vi "test_read_AB2504.vi"() -> ()   [LabVIEW 2015, in "Tausand AB1000.lvlib"]
uses:
  <instrlib>/Tausand AB1000/Tausand AB1000.lvlib
  <instrlib>/Tausand AB1000/Public/Controls/settings4ch.ctl
  <instrlib>/Tausand AB1000/Public/Controls/configMultipleCoincRing.ctl
  <instrlib>/Tausand AB1000/Public/Controls/counters4ch.ctl
  <instrlib>/Tausand AB1000/Public/Controls/deviceTypeRing.ctl
  <instrlib>/Tausand AB1000/Public/Controls/serialCommand.ctl
  <vilib>/Instr/_visa.llb/VISA Configure Serial Port (Instr).vi
panel:
  out "mode 3 timer":dbl format="%.1p"
  out "AB settg read timer":dbl format="%.1p"
  out "AB data read timer":dbl format="%.1p"
  out "porcentaje mal":dbl(slide) scale=0.0..100.0
  in  "ABlib on?":bool
  out "mode 2 timer":dbl format="%.1p"
  in  "mode3 on?":bool
  in  "mode2 on?":bool
  out "mode3 addr":u8[](array[numeric]) format="%.0x"
  out "mode3 data":u32[](array[numeric]) format="%.0x"
  in  "VISA resource name":refnum<visa-resource-name>
  in  "baud rate (115200)":u32=115200
  out "error out":errorcluster
  in  "device type":T1=1504 items=["any"=0, "AB1002"=1002, "AB1004"=1004, "AB1502"=1502, "AB1504"=1504, "AB1902"=1902, "AB1904"=1904]
  out "ID out":u32
  out "checksum ok?":bool
  in  "stop":bool
  out "porcentaje ok":dbl(slide) scale=0.0..100.0
  out "time left ms out":u32
  out "total ok":i32
  out "total try":i32
  out "output cluster 4ch":T2
  out "output cluster settings 4ch":T3 {"config_multiple_1" items=["ABC"=224, "ABD"=208, "ACD"=176, "BCD"=112, "ABCD"=240]; "sleep_D" max=100 step=5; "sleep_C" max=100 step=5; "sleep_B" max=100 step=5; "sleep_A" max=100 step=5; "delay_D" max=100 step=5; "delay_C" max=100 step=5; "delay_B" max=100 step=5; "delay_A" max=100 step=5; "coincidence_window" min=5 max=10000 step=5; "sampling" items=["1ms"=1, "2ms"=2, "3ms"=3, "4ms"=4, "5ms"=5, "6ms"=6, "7ms"=7, "8ms"=8, "9ms"=9, "10ms"=10, "11ms"=11, "12ms"=12, "13ms"=13, "14ms"=14, "15ms"=15, "16ms"=16, "17ms"=17, "18ms"=18, "19ms"=19, "20ms"=20, "21ms"=21, "22ms"=22, "23ms"=23, "24ms"=24, "25ms"=25, "26ms"=26, "27ms"=27, "28ms"=28, "29ms"=29, "30ms"=30, "31ms"=31, "32ms"=32, "33ms"=33, "34ms"=34, "35ms"=35, "36ms"=36, "37ms"=37, "38ms"=38, "39ms"=39, "40ms"=40, "41ms"=41, "42ms"=42, "43ms"=43, "44ms"=44, "45ms"=45, "46ms"=46, "47ms"=47, "48ms"=48, "49ms"=49, "50ms"=50, "51ms"=51, "52ms"=52, "53ms"=53, "54ms"=54, "55ms"=55, "56ms"=56, "57ms"=57, "58ms"=58, "59ms"=59, "60ms"=60, "61ms"=61, "62ms"=62, "63ms"=63, "64ms"=64, "65ms"=65, "66ms"=66, "67ms"=67, "68ms"=68, "69ms"=69, "70ms"=70, "71ms"=71, "72ms"=72, "73ms"=73, "74ms"=74, "75ms"=75, "76ms"=76, "77ms"=77, "78ms"=78, "79ms"=79, "80ms"=80, "81ms"=81, "82ms"=82, "83ms"=83, "84ms"=84, "85ms"=85, "86ms"=86, "87ms"=87, "88ms"=88, "89ms"=89, "90ms"=90, "91ms"=91, "92ms"=92, "93ms"=93, "94ms"=94, "95ms"=95, "96ms"=96, "97ms"=97, "98ms"=98, "99ms"=99, "100ms"=100, "110ms"=110, "120ms"=120, "130ms"=130, "140ms"=140, "150ms"=150, "160ms"=160, "170ms"=170, "180ms"=180, "190ms"=190, "200ms"=200, "210ms"=210, "220ms"=220, "230ms"=230, "240ms"=240, "250ms"=250, "260ms"=260, "270ms"=270, "280ms"=280, "290ms"=290, "300ms"=300, "310ms"=310, "320ms"=320, "330ms"=330, "340ms"=340, "350ms"=350, "360ms"=360, "370ms"=370, "380ms"=380, "390ms"=390, "400ms"=400, "410ms"=410, "420ms"=420, "430ms"=430, "440ms"=440, "450ms"=450, "460ms"=460, "470ms"=470, "480ms"=480, "490ms"=490, "500ms"=500, "510ms"=510, "520ms"=520, "530ms"=530, "540ms"=540, "550ms"=550, "560ms"=560, "570ms"=570, "580ms"=580, "590ms"=590, "600ms"=600, "610ms"=610, "620ms"=620, "630ms"=630, "640ms"=640, "650ms"=650, "660ms"=660, "670ms"=670, "680ms"=680, "690ms"=690, "700ms"=700, "710ms"=710, "720ms"=720, "730ms"=730, "740ms"=740, "750ms"=750, "760ms"=760, "770ms"=770, "780ms"=780, "790ms"=790, "800ms"=800, "810ms"=810, "820ms"=820, "830ms"=830, "840ms"=840, "850ms"=850, "860ms"=860, "870ms"=870, "880ms"=880, "890ms"=890, "900ms"=900, "910ms"=910, "920ms"=920, "930ms"=930, "940ms"=940, "950ms"=950, "960ms"=960, "970ms"=970, "980ms"=980, "990ms"=990, "1,0s"=1000, "1,1s"=1100, "1,2s"=1200, "1,3s"=1300, "1,4s"=1400, "1,5s"=1500, "1,6s"=1600, "1,7s"=1700, "1,8s"=1800, "1,9s"=1900, "2,0s"=2000, "2,1s"=2100, "2,2s"=2200, "2,3s"=2300, "2,4s"=2400, "2,5s"=2500, "2,6s"=2600, "2,7s"=2700, "2,8s"=2800, "2,9s"=2900, "3,0s"=3000, "3,1s"=3100, "3,2s"=3200, "3,3s"=3300, "3,4s"=3400, "3,5s"=3500, "3,6s"=3600, "3,7s"=3700, "3,8s"=3800, "3,9s"=3900, "4,0s"=4000, "4,1s"=4100, "4,2s"=4200, "4,3s"=4300, "4,4s"=4400, "4,5s"=4500, "4,6s"=4600, "4,7s"=4700, "4,8s"=4800, "4,9s"=4900, "5,0s"=5000, "5,1s"=5100, "5,2s"=5200, "5,3s"=5300, "5,4s"=5400, "5,5s"=5500, "5,6s"=5600, "5,7s"=5700, "5,8s"=5800, "5,9s"=5900, "6,0s"=6000, "6,1s"=6100, "6,2s"=6200, "6,3s"=6300, "6,4s"=6400, "6,5s"=6500, "6,6s"=6600, "6,7s"=6700, "6,8s"=6800, "6,9s"=6900, "7,0s"=7000, "7,1s"=7100, "7,2s"=7200, "7,3s"=7300, "7,4s"=7400, "7,5s"=7500, "7,6s"=7600, "7,7s"=7700, "7,8s"=7800, "7,9s"=7900, "8,0s"=8000, "8,1s"=8100, "8,2s"=8200, "8,3s"=8300, "8,4s"=8400, "8,5s"=8500, "8,6s"=8600, "8,7s"=8700, "8,8s"=8800, "8,9s"=8900, "9,0s"=9000, "9,1s"=9100, "9,2s"=9200, "9,3s"=9300, "9,4s"=9400, "9,5s"=9500, "9,6s"=9600, "9,7s"=9700, "9,8s"=9800, "9,9s"=9900, "10s"=10000, "11s"=11000, "12s"=12000, "13s"=13000, "14s"=14000, "15s"=15000, "16s"=16000, "17s"=17000, "18s"=18000, "19s"=19000, "20s"=20000, "21s"=21000, "22s"=22000, "23s"=23000, "24s"=24000, "25s"=25000, "26s"=26000, "27s"=27000, "28s"=28000, "29s"=29000, "30s"=30000, "31s"=31000, "32s"=32000, "33s"=33000, "34s"=34000, "35s"=35000, "36s"=36000, "37s"=37000, "38s"=38000, "39s"=39000, "40s"=40000, "41s"=41000, "42s"=42000, "43s"=43000, "44s"=44000, "45s"=45000, "46s"=46000, "47s"=47000, "48s"=48000, "49s"=49000, "50s"=50000, "51s"=51000, "52s"=52000, "53s"=53000, "54s"=54000, "55s"=55000, "56s"=56000, "57s"=57000, "58s"=58000, "59s"=59000, "60s"=60000, "61s"=61000, "62s"=62000, "63s"=63000, "64s"=64000, "65s"=65000, "66s"=66000, "67s"=67000, "68s"=68000, "69s"=69000, "70s"=70000, "71s"=71000, "72s"=72000, "73s"=73000, "74s"=74000, "75s"=75000, "76s"=76000, "77s"=77000, "78s"=78000, "79s"=79000, "80s"=80000, "81s"=81000, "82s"=82000, "83s"=83000, "84s"=84000, "85s"=85000, "86s"=86000, "87s"=87000, "88s"=88000, "89s"=89000, "90s"=90000, "91s"=91000, "92s"=92000, "93s"=93000, "94s"=94000, "95s"=95000, "96s"=96000, "97s"=97000, "98s"=98000, "99s"=99000, "100s"=100000, "110s"=110000, "120s"=120000, "130s"=130000, "140s"=140000, "150s"=150000, "160s"=160000, "170s"=170000, "180s"=180000, "190s"=190000, "200s"=200000, "210s"=210000, "220s"=220000, "230s"=230000, "240s"=240000, "250s"=250000, "260s"=260000, "270s"=270000, "280s"=280000, "290s"=290000, "300s"=300000, "310s"=310000, "320s"=320000, "330s"=330000, "340s"=340000, "350s"=350000, "360s"=360000, "370s"=370000, "380s"=380000, "390s"=390000, "400s"=400000, "410s"=410000, "420s"=420000, "430s"=430000, "440s"=440000, "450s"=450000, "460s"=460000, "470s"=470000, "480s"=480000, "490s"=490000, "500s"=500000, "510s"=510000, "520s"=520000, "530s"=530000, "540s"=540000, "550s"=550000, "560s"=560000, "570s"=570000, "580s"=580000, "590s"=590000, "600s"=600000, "610s"=610000, "620s"=620000, "630s"=630000, "640s"=640000, "650s"=650000, "660s"=660000, "670s"=670000, "680s"=680000, "690s"=690000, "700s"=700000, "710s"=710000, "720s"=720000, "730s"=730000, "740s"=740000, "750s"=750000, "760s"=760000, "770s"=770000, "780s"=780000, "790s"=790000, "800s"=800000, "810s"=810000, "820s"=820000, "830s"=830000, "840s"=840000, "850s"=850000, "860s"=860000, "870s"=870000, "880s"=880000, "890s"=890000, "900s"=900000, "910s"=910000, "920s"=920000, "930s"=930000, "940s"=940000, "950s"=950000, "960s"=960000, "970s"=970000, "980s"=980000, "990s"=990000, "1000s"=1000000]}
  out "mode2 addr":u8[](array[numeric]) format="%.0x"
  out "mode2 data":u32[](array[numeric]) format="%.0x"
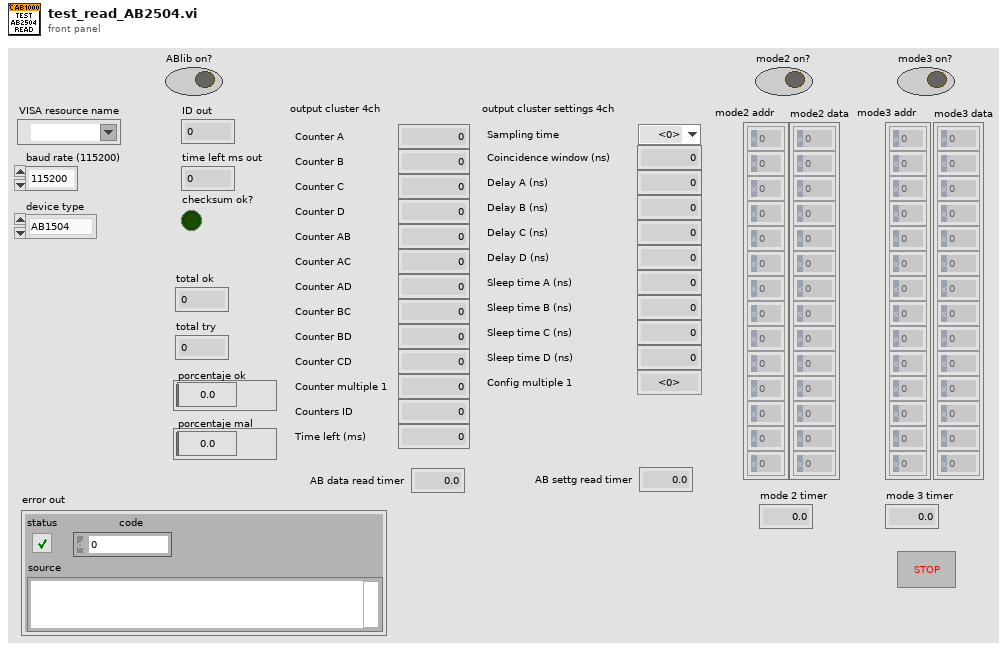
[diagram p1: front panel]
types:
  T1 = typedef "Tausand AB1000.lvlib/deviceTypeRing.ctl" = u16
  T2 = typedef "Tausand AB1000.lvlib/counters4ch.ctl" = cluster{"counter_A":u32, "counter_B":u32, "counter_C":u32, "counter_D":u32, "counter_AB":u32, "counter_AC":u32, "counter_AD":u32, "counter_BC":u32, "counter_BD":u32, "counter_CD":u32, "counter_multiple_1":u32, "counters_ID":u32, "time_left":u32}
  T3 = typedef "Tausand AB1000.lvlib/settings4ch.ctl" = cluster{"sampling":u32, "coincidence_window":u32, "delay_A":u32, "delay_B":u32, "delay_C":u32, "delay_D":u32, "sleep_A":u32, "sleep_B":u32, "sleep_C":u32, "sleep_D":u32, "config_multiple_1":T4}
  T4 = typedef "Tausand AB1000.lvlib/configMultipleCoincRing.ctl" = u16
  T5 = typedef "Tausand AB1000.lvlib/serialCommand.ctl" = u8
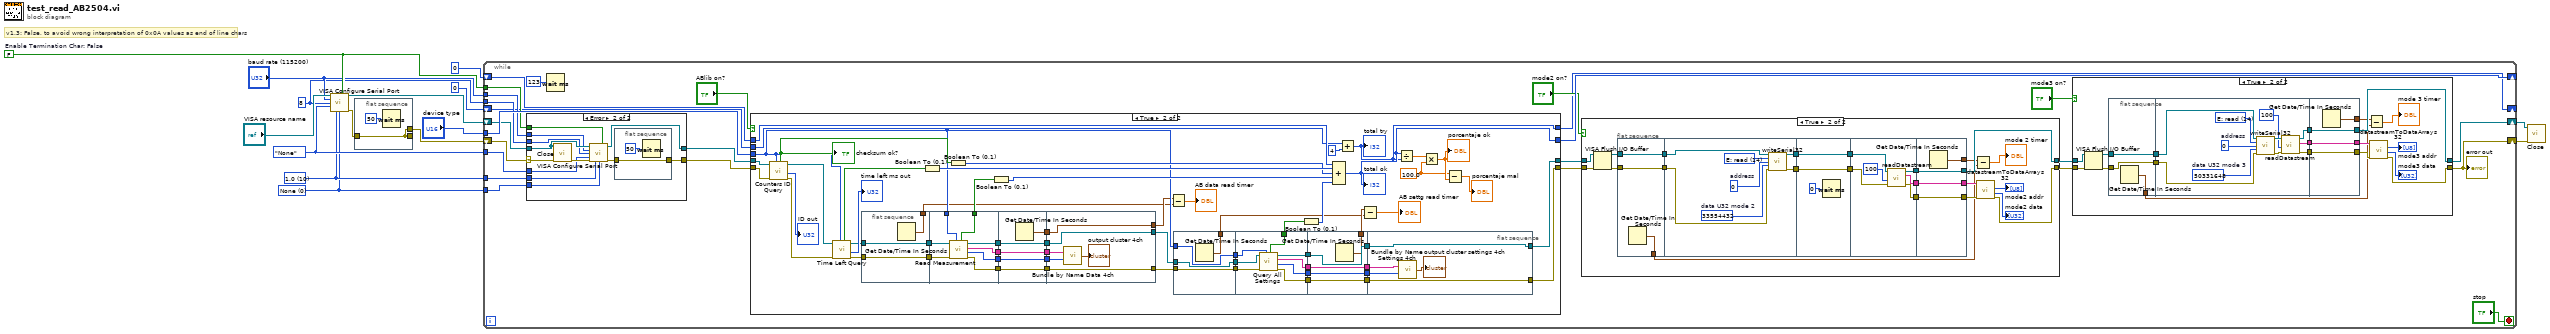
[diagram p0: block diagram]
diagram:
  w5 = u16 8 ("data bits (8)")
  w4 = enum16{"None", "Odd", "Even", "Mark", "Space"}."None" ("parity (0:none)")
  w3 = u16 10 items=["1.0"=10, "1.5"=15, "2.0"=20] ("stop bits (10: 1 bit)")
  w2 = u16 0 items=["None", "XON/XOFF", "RTS/CTS", "XON/XOFF & RTS/CTS", "DTR/DSR", "XON/XOFF & DTR/DSR"] ("flow control (0:none)")
  w7 = FALSE  # Enable Termination Char: False
  # "v1.3: False, to avoid wrong interpretation of 0x0A values as end of line chars"
  n1 = call-poly "VISA Configure Serial Port"("VISA resource name"="VISA resource name", "Enable Termination\nChar (T)"=w7, "baud rate (9600)"="baud rate (115200)", "data bits (8)"=w5, "parity (0:none)"=w4, "stop bits (10: 1 bit)"=w3, "flow control (0:none)"=w2) -> ("VISA resource name out"=w14:refnum<visa-resource-name>, "error out"=w13:errorcluster)  [unwired: 7 in]
  n2 = flat-sequence {
    tunnel: [w16] -> w11
    tunnel: [w16] -> _
    tunnel: w13 -> [w16]
    frame #0 {
      n3 = Wait (ms)(milliseconds to wait=u32 50) -> ()  [unwired: 1 out]
    }
  }
  n4 = while {
    tunnel: "device type" -> [w39]
    shift-right: [w21] -> w9
    shift-left: w11 -> [w31]
    shift-right: [w34] -> w10
    shift-left: w14 -> [w29]
    shift-right: [w41] -> _
    shift-left: 0 ("0, 1") -> [w42]
    tunnel: w7 -> [w27]
    tunnel: "baud rate (115200)" -> [w26]
    tunnel: w5 -> [w25]
    tunnel: w4 -> [w24]
    tunnel: w3 -> [w23]
    tunnel: w2 -> [w22]
    shift-right: [w18] -> _
    shift-left: 0 ("0, 1") -> [w19]
    stop <- "stop" stop-if-true
    n5 = case shown="Error" w31 {
      selector: w31 -> [w151 w161]
      tunnel: [w151 w153] -> w30
      tunnel: w29 -> [w150 w159]
      tunnel: [w150 w163] -> w28
      tunnel: w27 -> [_ w160]
      tunnel: w26 -> [_ w158]
      tunnel: w25 -> [_ w157]
      tunnel: w24 -> [_ w156]
      tunnel: w23 -> [_ w155]
      tunnel: w22 -> [_ w154]
      frame No Error {
      }
      frame Error {
        n6 = call <instrlib>:"Close.vi"("error in (no error)"=w161, "VISA resource name"=w159) -> ("error out"=w162:errorcluster)  [unwired: 9 in]
        n7 = call-poly "VISA Configure Serial Port"("VISA resource name"=w159, "Enable Termination\nChar (T)"=w160, "baud rate (9600)"=w158, "data bits (8)"=w157, "parity (0:none)"=w156, "error in (no error)"=w162, "stop bits (10: 1 bit)"=w155, "flow control (0:none)"=w154) -> ("VISA resource name out"=w163:refnum<visa-resource-name>, "error out"=w152:errorcluster)  [unwired: 6 in]
        n8 = flat-sequence {
          tunnel: [w165] -> w153
          tunnel: w152 -> [w165]
          frame #0 {
            n9 = Wait (ms)(milliseconds to wait=u32 50) -> ()  [unwired: 1 out]
          }
        }
      }
    }
    n10 = Wait (ms)(milliseconds to wait=u32 123) -> ()  [unwired: 1 out]
    n11 = case shown="True" "ABlib on?" {
      tunnel: w42 -> [w47 w101]
      tunnel: [w47 w99] -> w41
      tunnel: w39 -> [_ w93]
      tunnel: [w45 w92] -> w38
      tunnel: [w46 w91] -> w37
      tunnel: w30 -> [w45 w90]
      tunnel: w28 -> [w46 w89]
      tunnel: w19 -> [w44 w78]
      tunnel: [w44 w76] -> w18
      frame False {
      }
      frame True {
        w79 = 100.0 ("y")
        n12 = call <instrlib>:"Counters ID Query.vi"("device type"=w93, "error in (no error)"=w90, "VISA Refnum in"=w89) -> ("error out"=w88:errorcluster, "ID out"=→"ID out":u32, "VISA Refnum out"=w86:refnum<visa-resource-name>, "checksum ok?"=w105:bool)  [unwired: 5 in]
        "checksum ok?" <- w105
        n13 = call <instrlib>:"Time Left Query.vi"("device type"=w93, "error in (no error)"=w88, "VISA Refnum in"=w86) -> ("error out"=w84:errorcluster, "time left ms out"=→"time left ms out":u32, "VISA Refnum out"=w85:refnum<visa-resource-name>, "checksum ok?"=w104:bool)  [unwired: 5 in]
        n14 = flat-sequence {
          tunnel: w84 -> [w129]
          tunnel: w85 -> [w130]
          tunnel: [w130] -> w73
          tunnel: [w129] -> w72
          tunnel: [w128] -> w69
          tunnel: [w138] -> w96
          tunnel: w93 -> [w137]
          tunnel: [w134] -> w75
          tunnel: [w133] -> w74
          tunnel: w73 -> [w136]
          tunnel: w72 -> [w135]
          tunnel: [w132] -> w60
          tunnel: [w131] -> w57
          tunnel: w75 -> [w143]
          tunnel: w74 -> [w142]
          tunnel: [w143] -> w63
          tunnel: [w142] -> w62
          tunnel: [w141] -> w61
          tunnel: w60 -> [w140]
          tunnel: [w140] -> w59
          tunnel: [w139] -> w58
          tunnel: w57 -> [w139]
          tunnel: [w147] -> w70
          tunnel: [w148] -> w82
          tunnel: [w149] -> w83
          tunnel: w63 -> [w149]
          tunnel: w62 -> [w148]
          tunnel: w61 -> [w147]
          tunnel: w59 -> [w146]
          tunnel: w58 -> [w145]
          frame #0 {
            n15 = Get Date/Time In Seconds() -> (seconds since 1Jan1904=w128:timestamp)
          }
          frame #1 {
            n16 = call <instrlib>:"Read Measurement.vi"("device type"=w137, "error in (no error)"=w135, "VISA Refnum in"=w136) -> ("error out"=w133:errorcluster, "values"=w131:u32[], "labels"=w132:string[], "VISA Refnum out"=w134:refnum<visa-resource-name>, "checksum ok?"=w138:bool)  [unwired: 3 in, 1 out]
          }
          frame #2 {
            n17 = Get Date/Time In Seconds() -> (seconds since 1Jan1904=w141:timestamp)
          }
          frame #3 {
            n18 = call <instrlib>:"Bundle by Name Data 4ch.vi"("names"=w146, "values"=w145) -> ("output cluster 4ch"=→"output cluster 4ch":T2)  [unwired: 13 in]
          }
        }
        n19 = Boolean To (0,1)(Boolean=w104) -> (0, 1=w103:i16)
        n20 = Boolean To (0,1)(Boolean=w105) -> (0, 1=w102:i16)
        n21 = Boolean To (0,1)(Boolean=w96) -> (0, 1=w97:i16)
        n22 = Subtract(x=w70, y=w69) -> (x-y=→"AB data read timer":dbl)
        n23 = flat-sequence {
          tunnel: w82 -> [w107]
          tunnel: w83 -> [w108]
          tunnel: w93 -> [w109]
          tunnel: [w109] -> w68
          tunnel: [w108] -> w67
          tunnel: [w107] -> w66
          tunnel: [w106] -> w49
          tunnel: [w117] -> w95
          tunnel: w68 -> [w116]
          tunnel: w67 -> [w113]
          tunnel: w66 -> [w112]
          tunnel: [w115] -> w65
          tunnel: [w114] -> w64
          tunnel: [w111] -> w54
          tunnel: [w110] -> w51
          tunnel: w65 -> [w122]
          tunnel: w64 -> [w121]
          tunnel: [w122] -> w56
          tunnel: [w121] -> w55
          tunnel: w54 -> [w120]
          tunnel: [w120] -> w53
          tunnel: [w119] -> w52
          tunnel: w51 -> [w119]
          tunnel: [w118] -> w50
          tunnel: [w126] -> w91
          tunnel: [w127] -> w92
          tunnel: w56 -> [w127]
          tunnel: w55 -> [w126]
          tunnel: w53 -> [w124]
          tunnel: w52 -> [w123]
          frame #0 {
            n24 = Get Date/Time In Seconds() -> (seconds since 1Jan1904=w106:timestamp)
          }
          frame #1 {
            n25 = call <instrlib>:"Query All Settings.vi"("device type"=w116, "error in (no error)"=w112, "VISA Refnum in"=w113) -> ("error out"=w115:errorcluster, "values"=w110:u32[], "labels"=w111:string[], "VISA Refnum out"=w114:refnum<visa-resource-name>, "checksum ok?"=w117:bool)  [unwired: 4 in]
          }
          frame #2 {
            n26 = Get Date/Time In Seconds() -> (seconds since 1Jan1904=w118:timestamp)
          }
          frame #3 {
            n27 = call <instrlib>:"Bundle by Name Settings 4ch.vi"("names"=w124, "values"=w123) -> ("output cluster settings 4ch"=→"output cluster settings 4ch":T3)  [unwired: 13 in]
          }
        }
        n28 = Boolean To (0,1)(Boolean=w95) -> (0, 1=w94:i16)
        n29 = Compound Arithmetic op=ADD(w101, w103, w102, w97, w94) -> (w99:i32)
        "total ok" <- w99
        n30 = Add(x=w78, y=4) -> (x+y=w76:i32)
        "total try" <- w76
        n31 = Subtract(x=w50, y=w49) -> (x-y=→"AB settg read timer":dbl)
        n32 = Divide(x=w99, y=w76) -> (x/y=w98:dbl)
        n33 = Multiply(x=w98, y=w79) -> (x*y=w81:dbl)
        "porcentaje ok" <- w81
        n34 = Subtract(x=w79, y=w81) -> (x-y=→"porcentaje mal":dbl)
      }
    }
    n35 = case shown="True" "mode2 on?" {
      tunnel: w38 -> [w204 w221]
      tunnel: w37 -> [w205 w220]
      tunnel: [w204 w219] -> w36
      tunnel: [w205 w218] -> w35
      frame False {
      }
      frame True {
        n36 = VISA Flush I/O Buffer(VISA resource name=w220, error in (no error)=w221) -> (VISA resource name out=w226:refnum<visa-resource-name>, error out=w227:errorcluster)  [unwired: 1 in]
        n37 = flat-sequence {
          tunnel: w226 -> [w229]
          tunnel: w227 -> [w230]
          tunnel: [w230] -> w217
          tunnel: [w229] -> w216
          tunnel: [w228] -> w206
          tunnel: w217 -> [w237]
          tunnel: w216 -> [w236]
          tunnel: [w232] -> w210
          tunnel: [w231] -> w208
          tunnel: w210 -> [w240]
          tunnel: [w240] -> w209
          tunnel: w208 -> [w239]
          tunnel: [w239] -> w207
          tunnel: [w243] -> w213
          tunnel: [w241] -> w212
          tunnel: [w242] -> w211
          tunnel: w209 -> [w245]
          tunnel: w207 -> [w244]
          tunnel: [w248] -> w218
          tunnel: [w249] -> w224
          tunnel: [w250] -> w225
          tunnel: w213 -> [w250]
          tunnel: w212 -> [w249]
          tunnel: w211 -> [w248]
          tunnel: [w247] -> w215
          frame #0 {
            n38 = Get Date/Time In Seconds() -> (seconds since 1Jan1904=w228:timestamp)
          }
          frame #1 {
            w233 = u8 0  # address
            w234 = u32 33554432  # data U32 mode 2
            w235 = T5 14 items=["0", "1", "2", "3", "4", "5", "6", "7", "8", "9", "A", "B", "C", "D", "E: read", "F: write"] ("command (E: read)")
            n39 = call <instrlib>:"writeSerial32.vi"("VISA Refnum in"=w236, "command (E: read)"=w235, "address"=w233, "data U32 (0)"=w234, "error in (no error)"=w237) -> ("VISA Refnum out"=w232:refnum<visa-resource-name>, "error out"=w231:errorcluster)  [unwired: 9 in]
          }
          frame #2 {
            n40 = Wait (ms)(milliseconds to wait=u32 0) -> ()  [unwired: 1 out]
          }
          frame #3 {
            n41 = call <instrlib>:"readDatastream.vi"("error in (no error)"=w244, "Timeout (10000 ms)"=u32 100, "VISA Refnum in"=w245) -> ("error out"=w243:errorcluster, "string out"=w241:string, "VISA Refnum out"=w242:refnum<visa-resource-name>)  [unwired: 4 in, 2 out]
          }
          frame #4 {
            n42 = Get Date/Time In Seconds() -> (seconds since 1Jan1904=w247:timestamp)
          }
        }
        n43 = Subtract(x=w215, y=w206) -> (x-y=→"mode 2 timer":dbl)
        n44 = call <instrlib>:"datastreamToDataArrays32.vi"("error in (no error)"=w225, "input string"=w224) -> ("error out"=w219:errorcluster, "data32 out"=→"mode2 data":u32[], "addresses out"=→"mode2 addr":u8[])  [unwired: 5 in, 2 out]
      }
    }
    n45 = case shown="True" "mode3 on?" {
      tunnel: w36 -> [w166 w179]
      tunnel: [w166 w178] -> w21
      tunnel: w35 -> [w167 w177]
      tunnel: [w167 w176] -> w34
      frame False {
      }
      frame True {
        n46 = VISA Flush I/O Buffer(VISA resource name=w177, error in (no error)=w179) -> (VISA resource name out=w181:refnum<visa-resource-name>, error out=w180:errorcluster)  [unwired: 1 in]
        n47 = flat-sequence {
          tunnel: w180 -> [w187]
          tunnel: w181 -> [w188]
          tunnel: [w188] -> w172
          tunnel: [w187] -> w171
          tunnel: [w186] -> w168
          tunnel: [w195] -> w175
          tunnel: [w194] -> w174
          tunnel: [w190] -> w173
          tunnel: w172 -> [w192]
          tunnel: w171 -> [w191]
          tunnel: [w201] -> w176
          tunnel: [w202] -> w182
          tunnel: [w203] -> w183
          tunnel: w175 -> [w203]
          tunnel: w174 -> [w202]
          tunnel: w173 -> [w201]
          tunnel: [w200] -> w169
          frame #0 {
            n48 = Get Date/Time In Seconds() -> (seconds since 1Jan1904=w186:timestamp)
          }
          frame #1 {
            w199 = u8 0  # address
            w198 = u32 50331648  # data U32 mode 3
            w193 = T5 14 items=["0", "1", "2", "3", "4", "5", "6", "7", "8", "9", "A", "B", "C", "D", "E: read", "F: write"] ("command (E: read)")
            n49 = call <instrlib>:"writeSerial32.vi"("VISA Refnum in"=w192, "command (E: read)"=w193, "address"=w199, "data U32 (0)"=w198, "error in (no error)"=w191) -> ("VISA Refnum out"=w196:refnum<visa-resource-name>, "error out"=w197:errorcluster)  [unwired: 9 in]
            n50 = call <instrlib>:"readDatastream.vi"("error in (no error)"=w197, "Timeout (10000 ms)"=u32 100, "VISA Refnum in"=w196) -> ("error out"=w194:errorcluster, "string out"=w195:string, "VISA Refnum out"=w190:refnum<visa-resource-name>)  [unwired: 4 in, 2 out]
          }
          frame #2 {
            n51 = Get Date/Time In Seconds() -> (seconds since 1Jan1904=w200:timestamp)
          }
        }
        n52 = Subtract(x=w169, y=w168) -> (x-y=→"mode 3 timer":dbl)
        n53 = call <instrlib>:"datastreamToDataArrays32.vi"("error in (no error)"=w182, "input string"=w183) -> ("error out"=w178:errorcluster, "data32 out"=→"mode3 data":u32[], "addresses out"=→"mode3 addr":u8[])  [unwired: 5 in, 2 out]
      }
    }
    "error out" <- w21
  }
  n54 = call <instrlib>:"Close.vi"("error in (no error)"=w9, "VISA resource name"=w10) -> ()  [unwired: 9 in, 1 out]
